vi "rebuildMagBits.vi"(8 "error in (no error)":errorcluster, 11 "ByteArrayIn":u8[](array[numeric])) -> (0 "error out":errorcluster, 3 "rawBits":cluster{u16, u16, u16, u16})   [LabVIEW 2017, in "externalAquisition.lvlib"]
doc: "This VI rebuilds the sensor data into raw bits as measured by the teensy."
uses:
  externalAquisition.lvlib
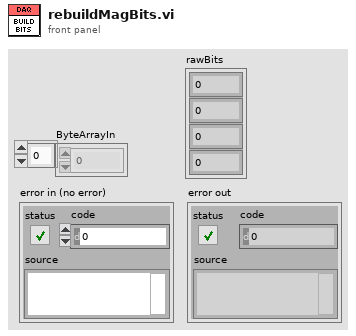
[diagram p1: front panel]
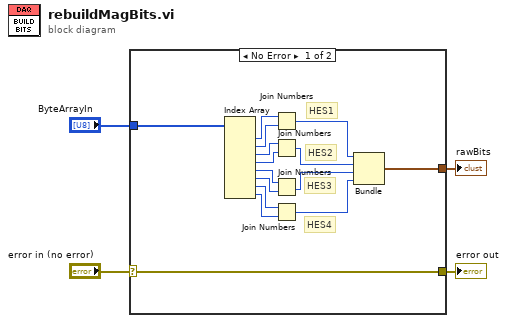
[diagram p0: block diagram]
diagram:
  n1 = case shown="No Error" "error in (no error)" {
    selector: "error in (no error)" -> [w10 w20]
    tunnel: [w10 w20] -> w3
    tunnel: "ByteArrayIn" -> [w19 _]
    tunnel: [w5 _] -> w1
    frame No Error {
      # "HES4"
      # "HES3"
      # "HES2"
      # "HES1"
      n2 = Index Array(array=w19) -> (element #1=w18:u8, element #2=w17:u8, element #3=w16:u8, element #4=w15:u8, element #5=w14:u8, element #6=w13:u8, element #7=w12:u8, element #8=w11:u8)  [unwired: 8 in]
      n3 = Join Numbers(hi=w18, lo=w17) -> ((hi.lo)=w9:u16)
      n4 = Join Numbers(hi=w16, lo=w15) -> ((hi.lo)=w8:u16)
      n5 = Join Numbers(hi=w14, lo=w13) -> ((hi.lo)=w7:u16)
      n6 = Join Numbers(hi=w12, lo=w11) -> ((hi.lo)=w6:u16)
      n7 = Bundle(w9, w8, w7, w6) -> (w5:cluster{u16, u16, u16, u16})  [unwired: 1 in]
    }
    frame Error {
    }
  }
  "error out" <- w3
  "rawBits" <- w1
